vi "Engine - Diesel - Boost Actuation Host.vi"() -> ()   [LabVIEW 2015, in "ECS-Host.lvlib"]
uses:
  ECS-Host.lvlib
  <vilib>/addons/Software Calibration Management/XControls/TBL1D.xctl
panel:
  out "WgPsnStp":sgl caption="[%Open]"
  out "WgDutyCyc_TblOut":sgl caption="[%]"
  out "WgDutyCyc_Des":sgl caption="[%]"
  in  "WgDutyCyc_Tbl":cluster{"X":sgl[], "Y":sgl[]}(xcontrol)
  in  "WgPWM_E":bool
  in  "WgPWMFreq":sgl caption="[Hz]"
  in  "WgDutyCyc_ManE":bool
  in  "WgDutyCyc_Man":sgl caption="[%]"
  in  "WgDutyCyc_Min":sgl caption="[%]"
  in  "WgDutyCyc_Max":sgl caption="[%]"
  out "VGTPsnStp":sgl caption="[%Open]"
  out "VGTDutyCyc_TblOut":sgl caption="[%]"
  out "VGTDutyCyc_Des":sgl caption="[%]"
  in  "VGTDutyCyc_Tbl":cluster{"X":sgl[], "Y":sgl[]}(xcontrol)
  in  "VGTPWM_E":bool
  in  "VGTPWMFreq":sgl caption="[Hz]"
  in  "VGTDutyCyc_ManE":bool
  in  "VGTDutyCyc_Man":sgl caption="[%]"
  in  "VGTDutyCyc_Min":sgl caption="[%]"
  in  "VGTDutyCyc_Max":sgl caption="[%]"
  # "Variable Geometry Turbocharger (VGT) Actuator"
  # "Wastegate (Wg) Actuator"
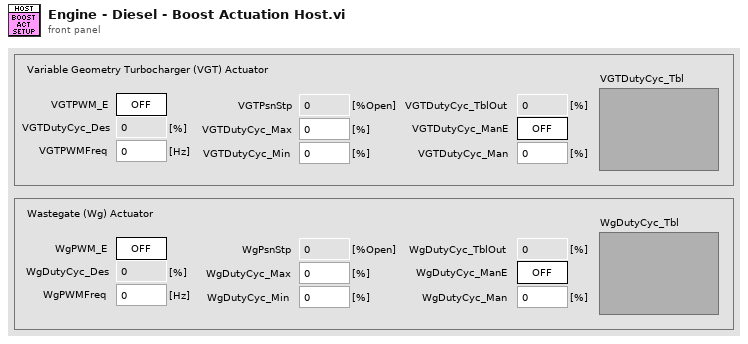
[diagram p1: front panel]
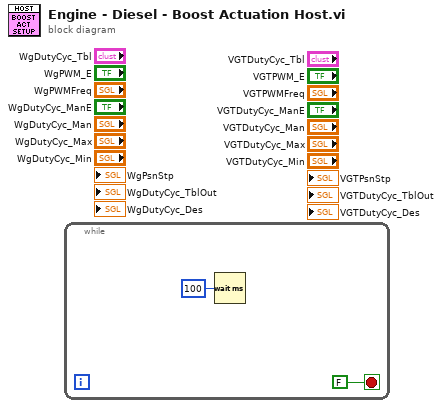
[diagram p0: block diagram]
diagram:
  n1 = while {
    stop <- FALSE stop-if-true
    n2 = Wait (ms)(milliseconds to wait=u32 100) -> ()  [unwired: 1 out]
  }
